vi "Remove Rows with Zeros 3D.vi"(1 "Index of 0 column":i32, 2 "Input Array":dbl[][][](array[numeric])) -> (0 "Rows with Zeros Removed":dbl[][][](array[numeric]))   [LabVIEW 2011]
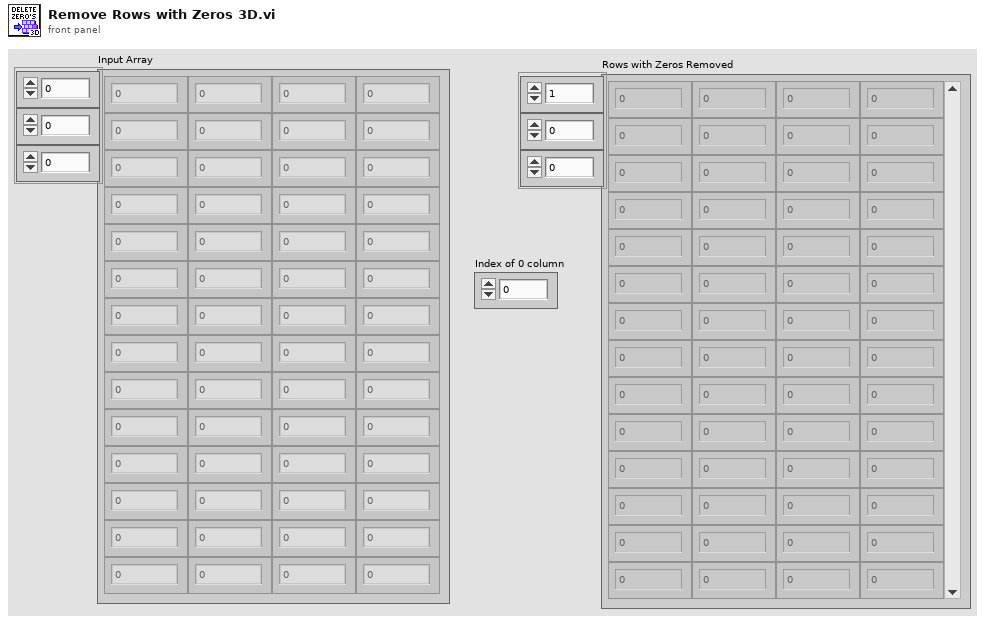
[diagram p1: front panel]
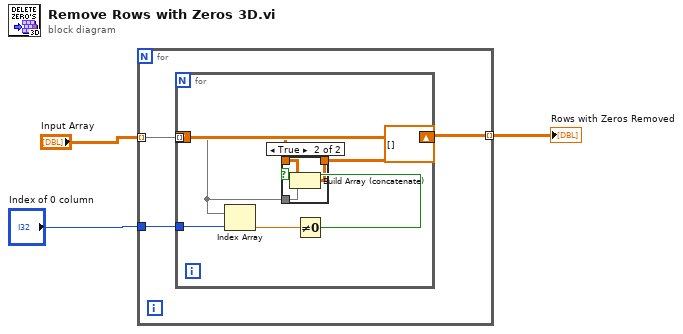
[diagram p0: block diagram]
diagram:
  n1 = for {
    tunnel: "Input Array" -> [w7] mode=indexing
    tunnel: [w6] -> w2 mode=indexing
    tunnel: "Index of 0 column" -> [w5]
    n2 = for {
      tunnel: w7 -> [w11] mode=indexing
      tunnel: w5 -> [w10]
      shift-right: [w8] -> w6
      shift-left: dbl[][] [] ("Input Array 2") -> [w9]
      n3 = Index Array(array=w11, index=w10) -> (element=w13:dbl)
      n4 = Not Equal To 0?(x=w13) -> (x != 0?=w12:bool)
      n5 = case shown="True" w12 {
        tunnel: w9 -> [w14 w16]
        tunnel: w11 -> [_ w15]
        tunnel: [w14 w17] -> w8
        frame False {
        }
        frame True {
          n6 = Build Array (concatenate)(w16, w15) -> (w17:dbl[][])
        }
      }
    }
  }
  "Rows with Zeros Removed" <- w2
